vi "Iterate.vi"(8 "error in (no error)":errorcluster, 10 "Iterator Settings":T1={"Prepare timeout (ms)"=200, "Iterate timeout (ms)"=50, "Conclude timeout (ms)"=200, "Iterate period (ms)"=200, "Number of iterations"=5, "Time before stop (ms)"=5, "Active Stop Conditions"={"Number of Iterations"=FALSE, "Time Elapsed"=FALSE, "Iteration Result"=FALSE}, "Prepare Msg"=refnum, "Iterate Msg"=refnum, "Conclude Msg"=refnum, "Iterations End Report"=refnum, "Message Priority (Normal)"=enum."Normal"}, 11 "Iterator Actor in":refnum<class "Iterator Actor.lvclass">) -> (0 "error out":errorcluster, 3 "Iterator Actor out":refnum<class "Iterator Actor.lvclass">)   [LabVIEW 2023, in "Iterator Actor.lvlib" / "Iterator Actor.lvclass"]
doc: "Iteratively calls the Iterate method of the Client. \nStops the iterations either by receiving the Stop signal, or by any of predefined Stop conditions."
uses:
  Iterator Actor.lvclass
  Abstract Iterator Actor/Iterator Settings.ctl
  Abstract Iterator Actor Messages/Iterator Report Iterations End Msg/Iterator Report Iterations End Msg.lvclass
  <vilib>/ActorFramework/Message/Message.lvclass
  Abstract Iterator Actor/Active Stop Conditions.ctl
  <vilib>/ActorFramework/Message Enqueuer/Message Priority.ctl
  C:/Program Files/National Instruments/LabVIEW 2023/vi.lib/ActorFramework/Actor/Actor.lvclass
  C:/Projects/Iterator Actor/Abstract Iterator Actor/Abstract Iterator Actor.lvclass
  Abstract Iterator Actor/Abstract Iterator Actor.lvclass/Abstract Iterator Actor.ctl
  <vilib>/ActorFramework/Actor/Actor.lvclass/Actor.ctl
  <vilib>/ActorFramework/Message Enqueuer/Message Enqueuer.lvclass/Message Enqueuer.ctl
  Abstract Iterator Actor/Stop Reason.ctl
  Iterator Actor Messages/Iterator Reply Msg/Iterator Reply Msg.lvclass
  C:/Program Files/National Instruments/LabVIEW 2023/vi.lib/ActorFramework/Message/Message.lvclass
  Iterator Actor Messages/Iterator Reply Msg/Iterator Reply Msg.lvclass/Iterator Reply Msg.ctl
  Abstract Iterator Actor/Read Stop Iterate Notifier.vi
  <vilib>/ActorFramework/Message Enqueuer/Init from Existing Queue.vi
  <vilib>/ActorFramework/Message Enqueuer/Enqueue.vi
  <vilib>/ActorFramework/Message Priority Queue/Priority Enqueue.vi
  <vilib>/Utility/error.llb/Error Cluster From Error Code.vi
  <vilib>/ActorFramework/Message Enqueuer/Message Enqueuer.lvclass
  <vilib>/ErrorRing/Error Ring.xnode
  Iterator Actor.lvclass/Iterator Actor.ctl
  <userlib>/_OpenG.lib/time/time.llb/openg_time.lvlib
  Abstract Iterator Actor Messages/Write Stop Reason Msg/Write Stop Reason Msg.lvclass
  <vilib>/ActorFramework/Actor/Actor.lvclass
  Abstract Iterator Actor/Abstract Iterator Actor.lvclass
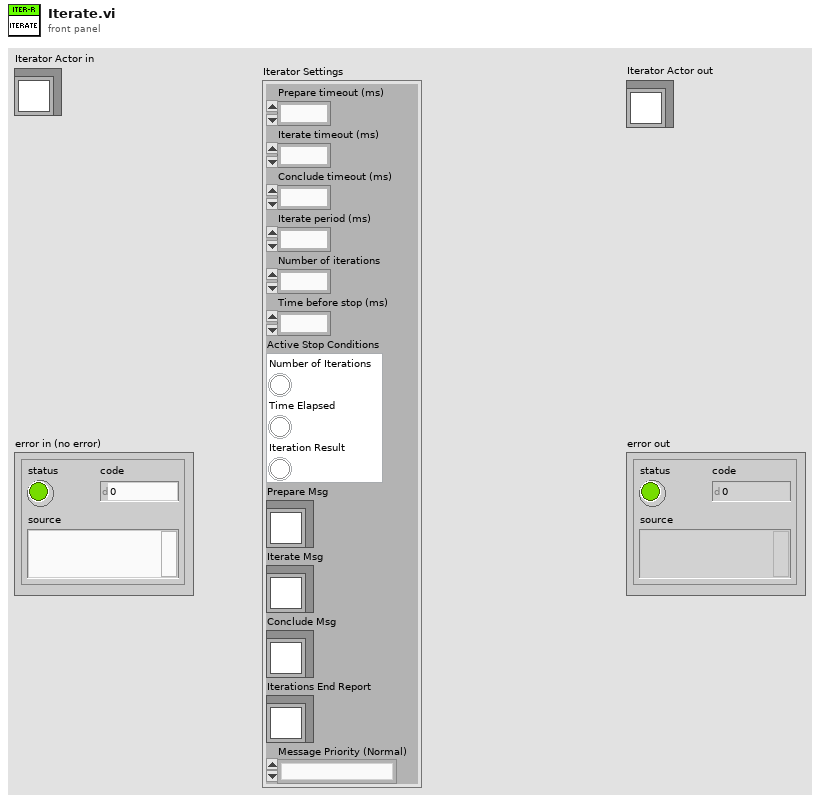
[diagram p1: front panel]
types:
  T1 = typedef "Iterator Actor.lvlib/Abstract Iterator Actor.lvclass/Iterator Settings.ctl" = cluster{"Prepare timeout (ms)":i32, "Iterate timeout (ms)":i32, "Conclude timeout (ms)":i32, "Iterate period (ms)":i32, "Number of iterations":i32, "Time before stop (ms)":i32, "Active Stop Conditions":T2, "Prepare Msg":refnum<class "Message.lvclass">, "Iterate Msg":refnum<class "Message.lvclass">, "Conclude Msg":refnum<class "Message.lvclass">, "Iterations End Report":refnum<class "Iterator Report Iterations End Msg.lvclass">, "Message Priority (Normal)":T3}
  T2 = typedef "Iterator Actor.lvlib/Abstract Iterator Actor.lvclass/Active Stop Conditions.ctl" = cluster{"Number of Iterations":bool, "Time Elapsed":bool, "Iteration Result":bool}
  T3 = typedef "Actor Framework.lvlib/Message Enqueuer.lvclass/Message Priority.ctl" = enum16{"Low", "Normal", "High"}
  T4 = typedef "Iterator Actor.lvlib/Abstract Iterator Actor.lvclass/Stop Reason.ctl" = enum16{"Number of Iterations", "Time Elapsed", "Stopped Internally", "Stopped Externally"}
  T5 = typedef "Iterator Actor.lvlib/Abstract Iterator Actor.lvclass/Stop Condition.ctl" = enum16{"None", "Number of Iterations", "Time Elapsed", "Iteration Result"}
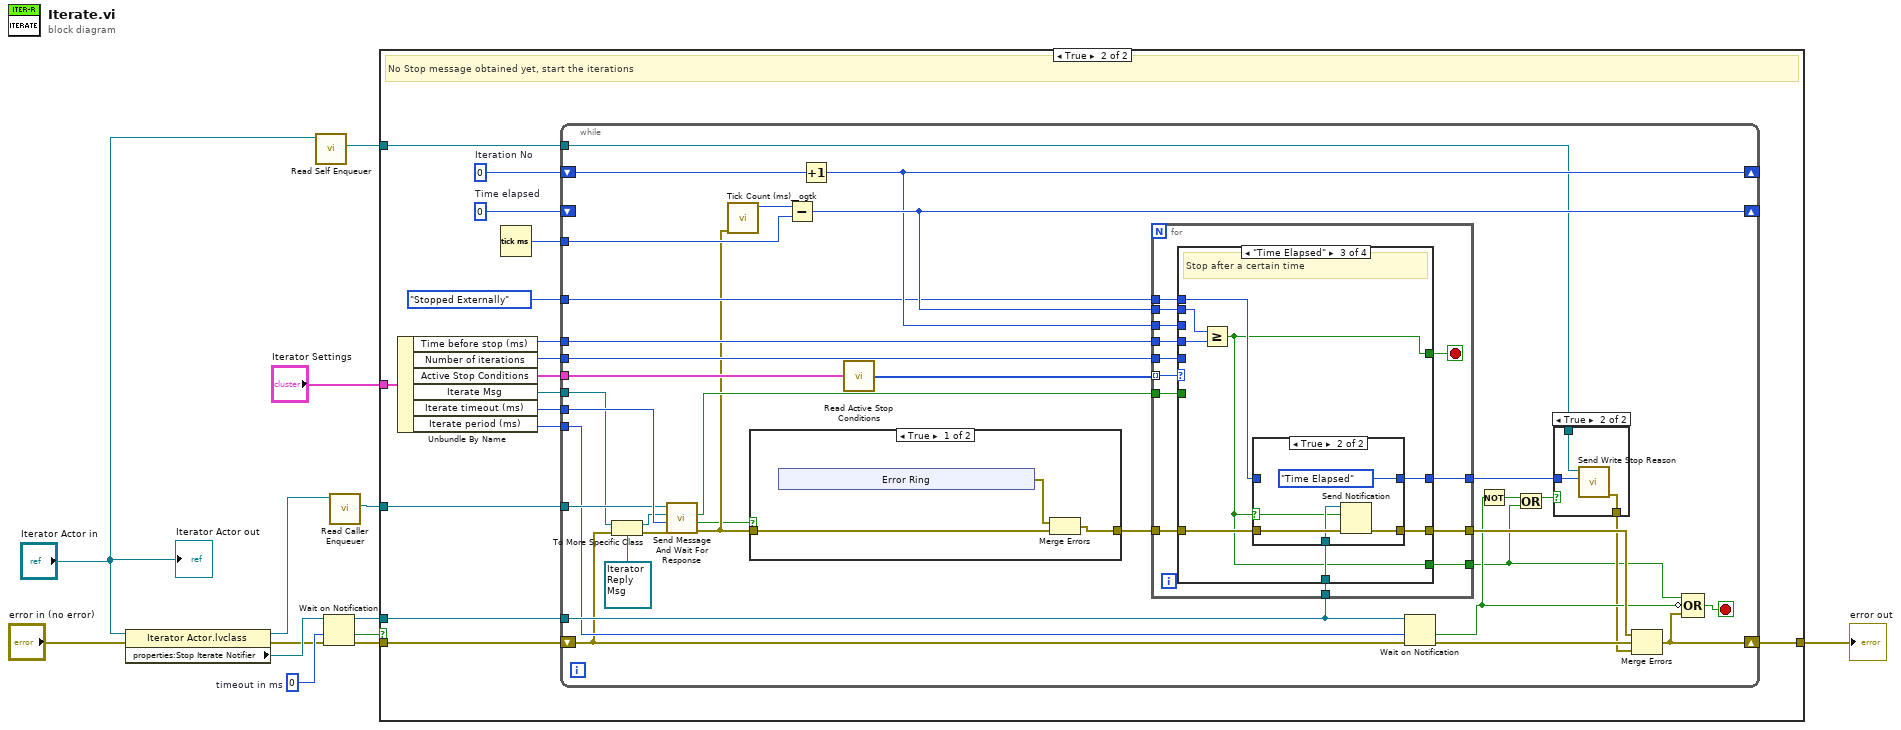
[diagram p0: block diagram]
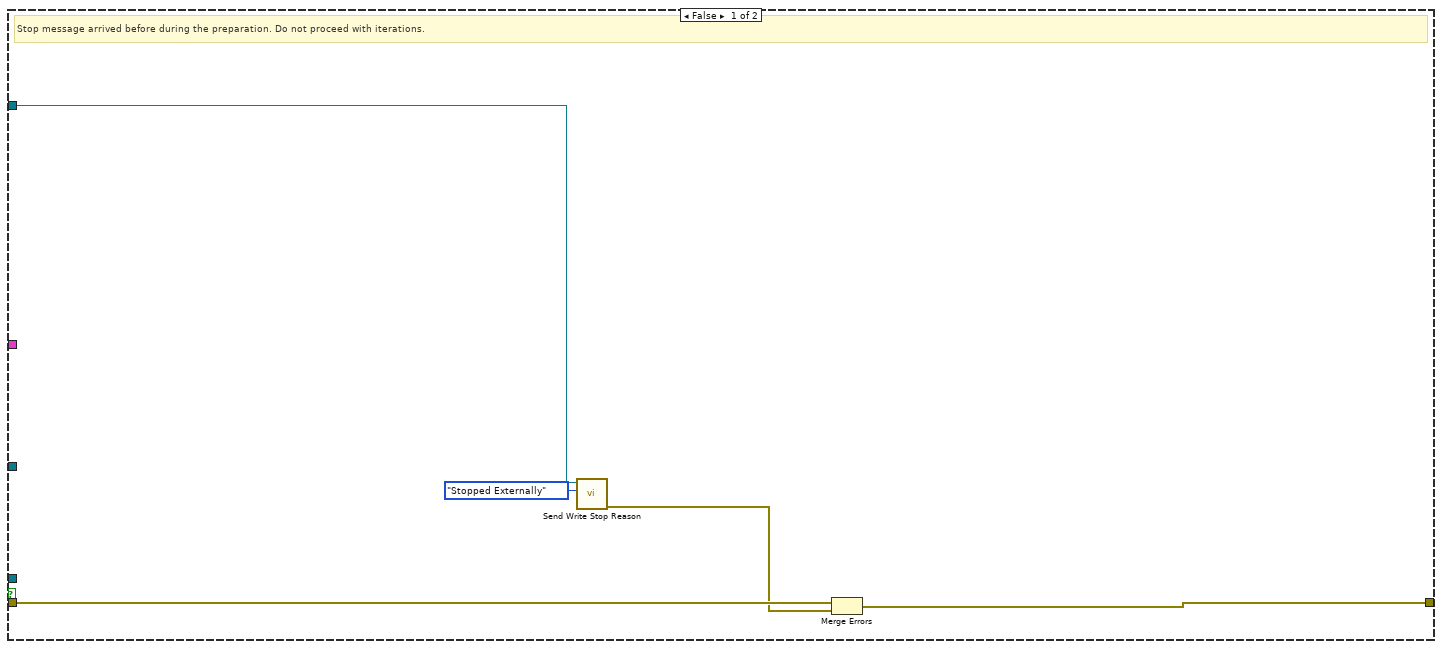
[diagram p2: hidden frame]
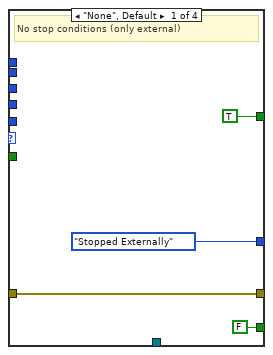
[diagram p4: hidden frame]
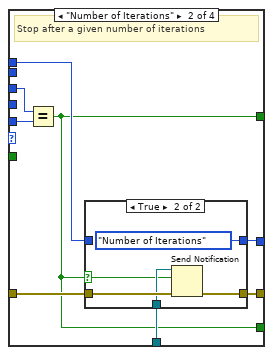
[diagram p5: hidden frame]
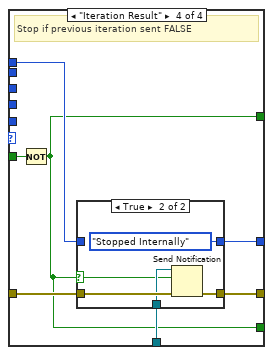
[diagram p8: hidden frame]
diagram:
  w8 = 0  # timeout in ms
  n1 = property class="Iterator Actor.lvclass"(reference="Iterator Actor in", error in="error in (no error)") -> (reference out=w1:refnum<class "Iterator Actor.lvclass">, error out=w2:errorcluster, "properties:Stop Iterate Notifier"=w3:refnum<notifier>)
  n2 = call <vilib>:"Read Self Enqueuer.vi"("Actor"="Iterator Actor in") -> ("Self Enqueuer"=w7:refnum<class "Message Enqueuer.lvclass">)  [unwired: 10 in]
  n3 = Wait on Notification(notifier=w3, timeout in ms (-1)=w8, error in (no error)=w2) -> (notifier out=w10:refnum<notifier>, timed out?=w9:bool, error out=w11:errorcluster)  [unwired: 1 in, 1 out]
  n4 = call <vilib>:"Read Caller Enqueuer.vi"("Actor"=w1) -> ("Caller Enqueuer"=w6:refnum<class "Message Enqueuer.lvclass">)  [unwired: 10 in]
  n5 = case shown="True" w9 {
    tunnel: "Iterator Settings" -> [_ w28]
    tunnel: w6 -> [_ w25]
    tunnel: [w15 w23] -> w12
    tunnel: w11 -> [w18 w22]
    tunnel: w10 -> [_ w21]
    tunnel: w7 -> [w17 w20]
    frame False {
      # "Stop message arrived before during the preparation. Do not proceed with iterations."
      n6 = call "Send Write Stop Reason.vi"("Stop Reason"=Stop_Reason."Stopped Externally", "Message Enqueuer in"=w17) -> ("error out"=w14:errorcluster)  [unwired: 8 in, 1 out]
      n7 = Merge Errors(w18, w14) -> (w15:errorcluster)
    }
    frame True {
      w24 = 0  # Iteration No
      w26 = u32 0  # Time elapsed
      # "No Stop message obtained yet, start the iterations"
      n8 = Unbundle By Name(w28) -> ("Time before stop (ms)"=w29:i32, "Number of iterations"=w30:i32, "Active Stop Conditions"=w31:T2, "Iterate Msg"=w32:refnum<class "Message.lvclass">, "Iterate timeout (ms)"=w33:i32, "Iterate period (ms)"=w34:i32)
      n9 = Tick Count (ms)() -> (millisecond timer value=w27:u32)
      n10 = while {
        tunnel: w32 -> [w42]
        tunnel: w33 -> [w68]
        tunnel: w34 -> [w53]
        shift-right: [w54] -> w23
        shift-left: w22 -> [w44]
        shift-right: [w58] -> _
        shift-left: w24 -> [w65]
        shift-right: [w59] -> _
        shift-left: w26 -> [_]
        tunnel: w31 -> [w47]
        tunnel: w30 -> [w64]
        tunnel: w29 -> [w63]
        tunnel: w27 -> [w60]
        tunnel: w25 -> [w57]
        tunnel: w21 -> [w55]
        tunnel: w20 -> [w52]
        tunnel: Stop_Reason."Stopped Externally" ("Stop Reason") -> [w48]
        stop <- w62 stop-if-true
        n11 = To More Specific Class(target class=refnum<class "Iterator Reply Msg.lvclass"> refnum ("Iterator Actor.lvlib:Iterator Reply Msg"), reference=w42, error in=w44) -> (specific class reference=w41:refnum<class "Iterator Reply Msg.lvclass">, error out=w45:errorcluster)
        n12 = call "Send Message And Wait For Response.vi"("error in (no error)"=w45, "timeout in ms (-1)"=w68, "Original Message"=w41, "Message Enqueuer in"=w57) -> ("error out"=w37:errorcluster, "timed out?"=w35:bool, "Reply"=w56:bool)  [unwired: 4 in, 1 out]
        n13 = call <userlib>:"Tick Count (ms)__ogtk.vi"("error in (no error)"=w37) -> ("millisecond timer value"=w61:u32)  [unwired: 9 in, 1 out]
        n14 = case shown="True" w35 {
          tunnel: w37 -> [w71 w76]
          tunnel: [w70 w76] -> w36
          frame True {
            n15 = xnode "Error Ring"() -> ("error out"=w69:errorcluster)
            n16 = Merge Errors(w69, w71) -> (w70:errorcluster)
          }
          frame False {
          }
        }
        n17 = Subtract(x=w61, y=w60) -> (x-y=w59:u32)
        n18 = Increment(x=w65) -> (x+1=w58:i32)
        n19 = call "Read Active Stop Conditions.vi"("Active Stop Conditions"=w47) -> ("Active Stop Conditions"=w46:T5[])
        n20 = for {
          tunnel: w46 -> [w88] mode=indexing
          tunnel: w64 -> [w87]
          tunnel: w63 -> [w86]
          tunnel: w59 -> [w84]
          tunnel: w58 -> [w83]
          tunnel: w56 -> [w82]
          tunnel: w55 -> [w81]
          tunnel: w36 -> [w85]
          tunnel: [w89] -> w66
          tunnel: w48 -> [w79]
          tunnel: [w80] -> w51
          tunnel: [w77] -> w39
          stop <- w78 stop-if-true
          n21 = case shown="\"Time Elapsed\"" w88 {
            tunnel: w85 -> [w93 w99 w116 w128]
            tunnel: [w93 w98 w115 w130] -> w89
            tunnel: w81 -> [_ w101 w114 w129]
            tunnel: w87 -> [_ w100 _ _]
            tunnel: w86 -> [_ _ w113 _]
            tunnel: w84 -> [_ _ w112 _]
            tunnel: w83 -> [_ w97 _ _]
            tunnel: w82 -> [_ _ _ w125]
            tunnel: [Stop_Reason."Stopped Externally" ("Stop Reason") w96 w111 w127] -> w80
            tunnel: w79 -> [_ w95 w110 w126]
            tunnel: [TRUE ("Reply") w94 w109 w124] -> w78
            tunnel: [FALSE w94 w109 w124] -> w77
            frame "None", Default {
              # "No stop conditions (only external)"
            }
            frame "Number of Iterations" {
              # "Stop after a given number of iterations"
              n22 = Equal?(x=w97, y=w100) -> (x = y?=w94:bool)
              n23 = case shown="True" w94 {
                selector: w94 -> [_ w104]
                tunnel: w101 -> [_ w106]
                tunnel: w99 -> [w103 w108]
                tunnel: [w103 w107] -> w98
                tunnel: [w102 Stop_Reason."Number of Iterations" ("Stop Reason")] -> w96
                tunnel: w95 -> [w102 _]
                frame False {
                }
                frame True {
                  n24 = Send Notification(notification=w104, notifier=w106, error in (no error)=w108) -> (error out=w107:errorcluster)  [unwired: 1 out]
                }
              }
            }
            frame "Time Elapsed" {
              # "Stop after a certain time"
              n25 = Greater Or Equal?(x=w112, y=w113) -> (x >= y?=w109:bool)
              n26 = case shown="True" w109 {
                selector: w109 -> [_ w120]
                tunnel: w114 -> [_ w121]
                tunnel: w116 -> [w118 w123]
                tunnel: [w118 w122] -> w115
                tunnel: [w117 Stop_Reason."Time Elapsed" ("Stop Reason")] -> w111
                tunnel: w110 -> [w117 _]
                frame False {
                }
                frame True {
                  n27 = Send Notification(notification=w120, notifier=w121, error in (no error)=w123) -> (error out=w122:errorcluster)  [unwired: 1 out]
                }
              }
            }
            frame "Iteration Result" {
              # "Stop if previous iteration sent FALSE"
              n28 = Not(x=w125) -> (.not. x?=w124:bool)
              n29 = case shown="True" w124 {
                selector: w124 -> [_ w134]
                tunnel: w129 -> [_ w135]
                tunnel: w128 -> [w132 w137]
                tunnel: [w132 w136] -> w130
                tunnel: [w131 Stop_Reason."Stopped Internally" ("Stop Reason")] -> w127
                tunnel: w126 -> [w131 _]
                frame False {
                }
                frame True {
                  n30 = Send Notification(notification=w134, notifier=w135, error in (no error)=w137) -> (error out=w136:errorcluster)  [unwired: 1 out]
                }
              }
            }
          }
        }
        n31 = Wait on Notification(notifier=w55, timeout in ms (-1)=w53, error in (no error)=w44) -> (timed out?=w50:bool, error out=w67:errorcluster)  [unwired: 1 in, 2 out]
        n32 = Not(x=w50) -> (.not. x?=w38:bool)
        n33 = Or(x=w38, y=w39) -> (x .or. y?=w40:bool)
        n34 = case shown="True" w40 {
          tunnel: w52 -> [_ w140]
          tunnel: w51 -> [_ w139]
          tunnel: [_ w138] -> w49
          frame False {
          }
          frame True {
            n35 = call "Send Write Stop Reason.vi"("Stop Reason"=w139, "Message Enqueuer in"=w140) -> ("error out"=w138:errorcluster)  [unwired: 8 in, 1 out]
          }
        }
        n36 = Merge Errors(w66, w67, w49) -> (w54:errorcluster)
        n37 = Compound Arithmetic op=OR(w39, invert w50, w54) -> (w62:bool)
      }
    }
  }
  "error out" <- w12
  "Iterator Actor out" <- "Iterator Actor in"
